vi "GET_IconTextClass.vi"(8 "error in (no error)":errorcluster, 11 "Icon.lvclass in":refnum<class "Icon.lvclass">) -> (0 "error out":errorcluster, 2 "Icon Framework.lvclass":refnum<class "Icon Framework.lvclass">, 3 "Icon.lvclass out":refnum<class "Icon.lvclass">)   [LabVIEW 2021, in "Icon.lvclass"]
doc: "Returns the Text Layer."
uses:
  Icon.lvclass
  Icon Framework/Icon Framework.lvclass
  Icon.lvclass/Icon.ctl
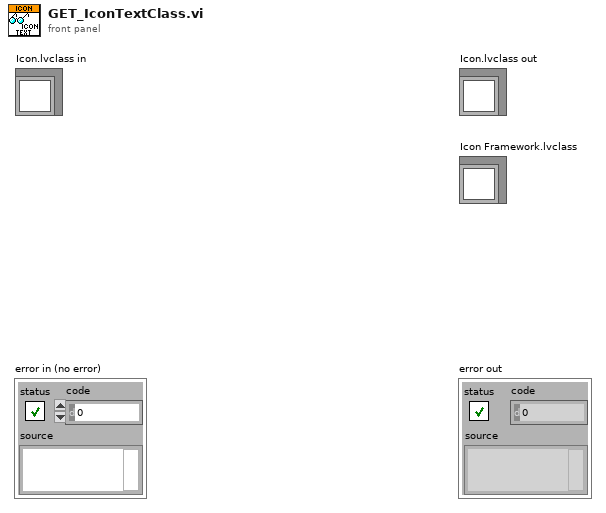
[diagram p1: front panel]
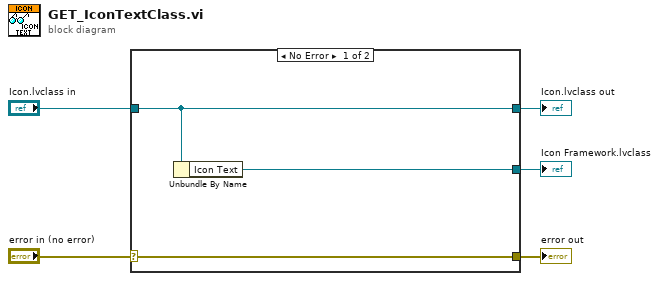
[diagram p0: block diagram]
diagram:
  n1 = case shown="No Error" "error in (no error)" {
    selector: "error in (no error)" -> [w8 w9]
    tunnel: [w8 w9] -> w4
    tunnel: [w7 w10] -> w2
    tunnel: "Icon.lvclass in" -> [w7 w10]
    tunnel: [w6 _] -> w1
    frame No Error {
      n2 = Unbundle By Name(w7) -> ("Icon Text"=w6:refnum<class "Icon Framework.lvclass">)
    }
    frame Error {
    }
  }
  "error out" <- w4
  "Icon.lvclass out" <- w2
  "Icon Framework.lvclass" <- w1
